vi "Get Depth Image.vi"(8 "error in (no error)":errorcluster, 9 "Wait For Next Image?":bool=TRUE, 11 "Reference In":T1) -> (0 "error out":errorcluster, 1 "Depth Image Pixels (U16)":u16[][](array[numeric]), 2 "Depth Image":T2(plugin-control), 3 "Reference Out":T1)   [LabVIEW 2011]
uses:
  <vilib>/vision/Image Controls.llb/IMAQ Image.ctl
  Microsoft.Research.Kinect
panel:
  out "Image Is New?":bool
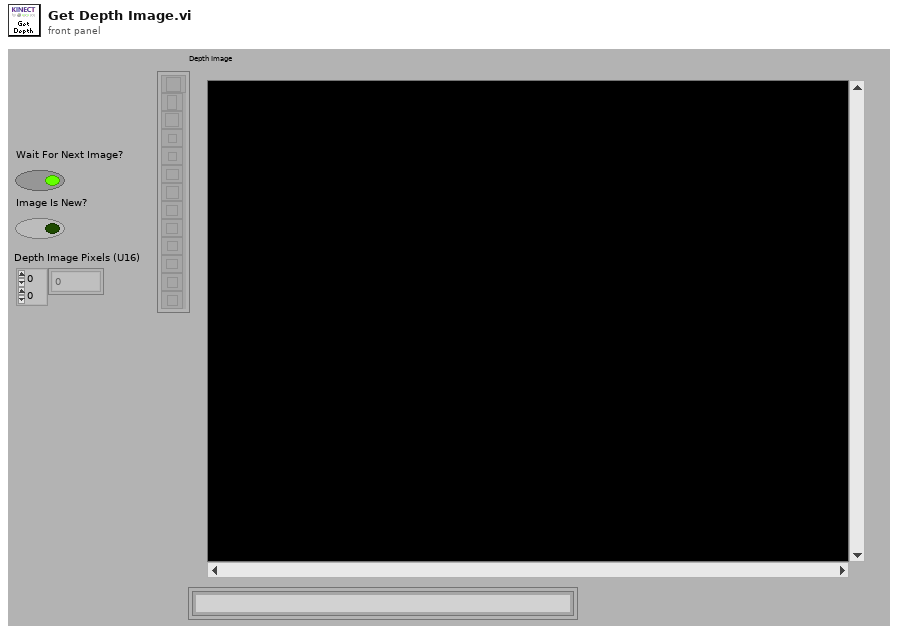
[diagram p1: front panel]
types:
  T1 = cluster{cluster{"queue out":refnum<queue>, "queue out":refnum<queue>}, cluster{"new reference":refnum<k24>, "DepthStream":refnum<k24>, "VideoStream":refnum<k24>, "Event Callback":refnum<k27>, "Event Callback":refnum<k27>}}
  T2 = typedef "IMAQ Image.ctl" = refnum<image>
  T3 = cluster{"queue out":refnum<queue>, "queue out":refnum<queue>}
  T4 = typedef "Image Type" = u32
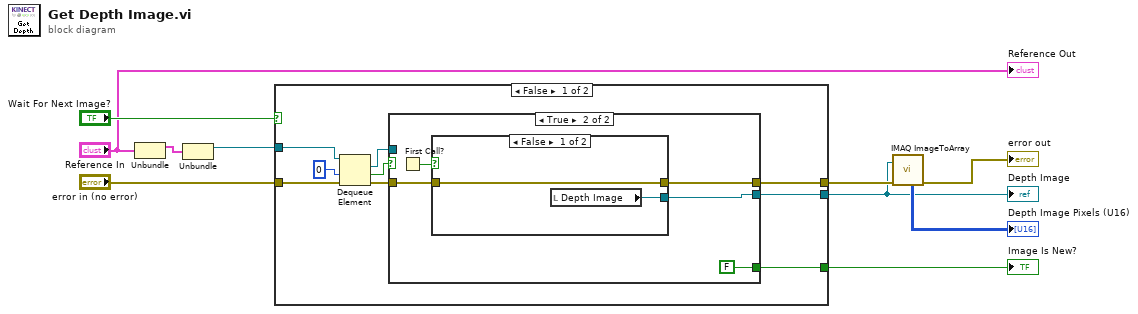
[diagram p0: block diagram]
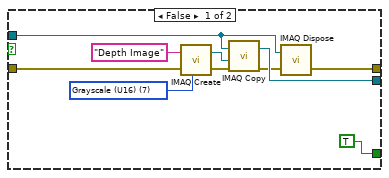
[diagram p2: hidden frame]
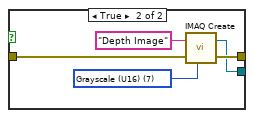
[diagram p3: hidden frame]
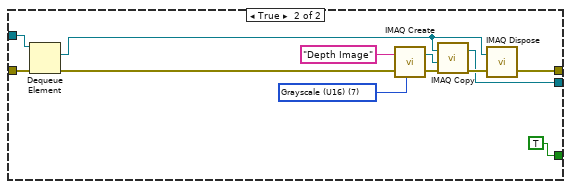
[diagram p4: hidden frame]
diagram:
  n1 = Unbundle("Reference In") -> (w2:T3)  [unwired: 1 out]
  n2 = Unbundle(w2) -> ("queue out"=w1:refnum<queue>)  [unwired: 1 out]
  n3 = case shown="False" "Wait For Next Image?" {
    tunnel: "error in (no error)" -> [w15 w53]
    tunnel: [w17 w42] -> w5
    tunnel: [w18 w43] -> w6
    tunnel: [w19 TRUE] -> w9
    tunnel: w1 -> [w16 w51]
    frame False {
      n4 = Dequeue Element(queue=w16, timeout in ms (-1)=0, error in (no error)=w15) -> (element=w11:T2, timed out?=w12:bool, error out=w14:errorcluster)  [unwired: 1 out]
      n5 = case shown="True" w12 {
        tunnel: [w25 w32] -> w17
        tunnel: w14 -> [w20 w31]
        tunnel: [w22 w30] -> w18
        tunnel: [TRUE FALSE] -> w19
        tunnel: w11 -> [w21 _]
        frame False {
          w24 = T4 7 items=["Grayscale (U8)", "Grayscale (I16)", "Grayscale (SGL)", "Complex (CSG)", "RGB (U32)", "HSL (U32)", "RGB (U64)", "Grayscale (U16)"] ("Image Type")
          n6 = call "IMAQ Create"("Image Name"="Depth Image", "Image Type"=w24, "error in (no error)"=w20) -> ("New Image"=w27:T2, "error out"=w26:errorcluster)  [unwired: 2 in]
          n7 = call "IMAQ Copy"("error in (no error)"=w26, "Image Dst"=w27, "Image Src"=w21) -> ("error out"=w23:errorcluster, "Image Dst Out"=w25:T2)  [unwired: 3 in]
          n8 = call "IMAQ Dispose"("Image"=w21, "error in (no error)"=w23) -> ("error out"=w22:errorcluster)  [unwired: 4 in]
        }
        frame True {
          n9 = First Call?() -> (First Call?: T/F=w33:bool)
          n10 = case shown="False" w33 {
            tunnel: [w36 w37] -> w32
            tunnel: w31 -> [w35 w39]
            tunnel: [w35 w38] -> w30
            frame False {
              n11 = local read "Depth Image"() -> (w36:T2)
            }
            frame True {
              w40 = T4 7 items=["Grayscale (U8)", "Grayscale (I16)", "Grayscale (SGL)", "Complex (CSG)", "RGB (U32)", "HSL (U32)", "RGB (U64)", "Grayscale (U16)"] ("Image Type")
              n12 = call "IMAQ Create"("Image Name"="Depth Image", "Image Type"=w40, "error in (no error)"=w39) -> ("New Image"=w37:T2, "error out"=w38:errorcluster)  [unwired: 2 in]
            }
          }
        }
      }
    }
    frame True {
      w46 = T4 7 items=["Grayscale (U8)", "Grayscale (I16)", "Grayscale (SGL)", "Complex (CSG)", "RGB (U32)", "HSL (U32)", "RGB (U64)", "Grayscale (U16)"] ("Image Type")
      n13 = Dequeue Element(queue=w51, error in (no error)=w53) -> (element=w45:T2, error out=w49:errorcluster)  [unwired: 1 in, 2 out]
      n14 = call "IMAQ Create"("Image Name"="Depth Image", "Image Type"=w46, "error in (no error)"=w49) -> ("New Image"=w48:T2, "error out"=w47:errorcluster)  [unwired: 2 in]
      n15 = call "IMAQ Copy"("error in (no error)"=w47, "Image Dst"=w48, "Image Src"=w45) -> ("error out"=w44:errorcluster, "Image Dst Out"=w42:T2)  [unwired: 3 in]
      n16 = call "IMAQ Dispose"("Image"=w45, "error in (no error)"=w44) -> ("error out"=w43:errorcluster)  [unwired: 4 in]
    }
  }
  "Depth Image" <- w5
  "Image Is New?" <- w9
  n17 = call "IMAQ ImageToArray"("error in (no error)"=w6, "Image"=w5) -> ("Image Pixels (U16)"=→"Depth Image Pixels (U16)":u16[][], "error out"=→"error out":errorcluster)  [unwired: 2 in, 3 out]
  "Reference Out" <- "Reference In"
